vi "secondsToTime.vi"(11 "Time input (ms)":dbl) -> (3 "Time Stamp":string)   [LabVIEW 2021]
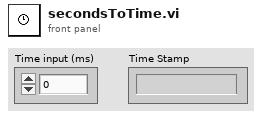
[diagram p1: front panel]
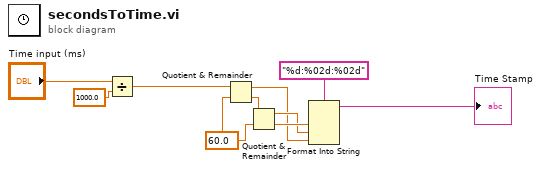
[diagram p0: block diagram]
diagram:
  w10 = 60.0 ("y")
  n1 = Divide(x="Time input (ms)", y=1000.0 ("x")) -> (x/y=w2:dbl)
  n2 = Quotient & Remainder(x=w2, y=w10) -> (x-y*floor(x/y)=w4:dbl, floor(x/y)=w3:dbl)
  n3 = Quotient & Remainder(x=w3, y=w10) -> (x-y*floor(x/y)=w5:dbl, floor(x/y)=w6:dbl)
  n4 = Format Into String(format string="%d:%02d:%02d", w6, w5, w4) -> (resulting string=→"Time Stamp":string)  [unwired: 2 in, 1 out]
